vi "retrieve_graph_data.vi"(1 "Time":sgl, 2 "Data Cluster":T1, 3 "handle":i32) -> (0 "output cluster":T1)   [LabVIEW 2015]
uses:
  MWT.dll
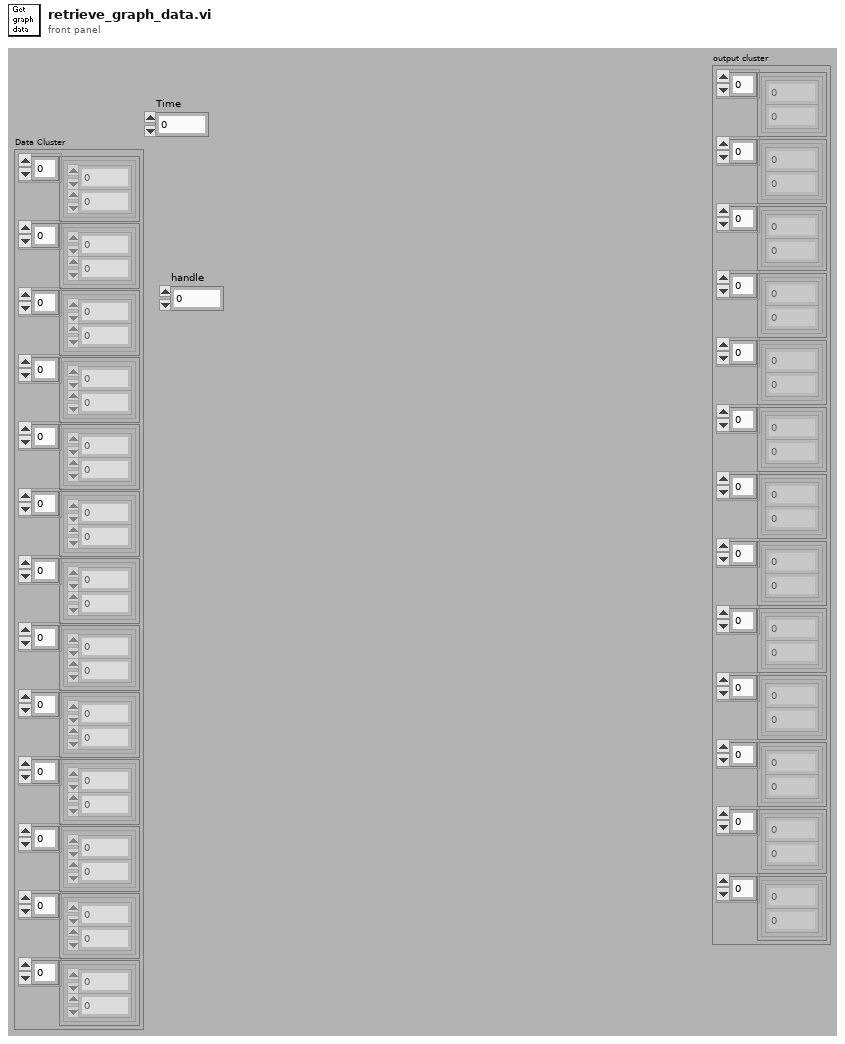
[diagram p1: front panel]
types:
  T1 = cluster{cluster{sgl, sgl}[], cluster{sgl, sgl}[], cluster{sgl, sgl}[], cluster{sgl, sgl}[], cluster{sgl, sgl}[], cluster{sgl, sgl}[], cluster{sgl, sgl}[], cluster{sgl, sgl}[], cluster{sgl, sgl}[], cluster{sgl, sgl}[], cluster{sgl, sgl}[], cluster{sgl, sgl}[], cluster{sgl, sgl}[]}
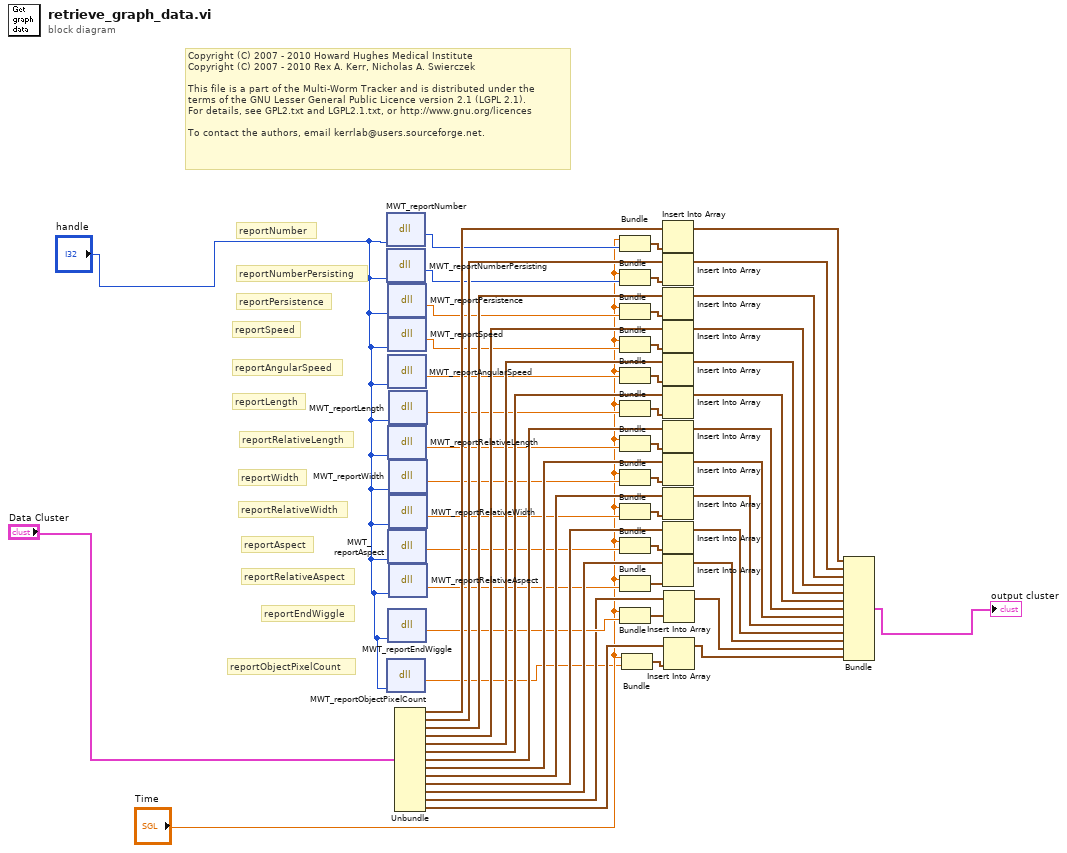
[diagram p0: block diagram]
diagram:
  # "reportObjectPixelCount"
  # "Copyright (C) 2007 - 2010 Howard Hughes Medical Institute\nCopyright (C) 2007 - 2010 Rex A. Kerr, Nicholas A. Swierczek\n \nThis file is a part of the Multi-Worm Tracker and is distributed under the\nterms of the GNU Lesser General Public Licence version 2.1 (LGPL 2.1).\nFor details, see GPL2.txt and LGPL2.1.txt, or http://www.gnu.org/licences\n \nTo contact the authors, email kerrlab@users.sourceforge.net."
  # "reportEndWiggle"
  # "reportRelativeAspect"
  # "reportAspect"
  # "reportRelativeWidth"
  # "reportWidth"
  # "reportRelativeLength"
  # "reportLength"
  # "reportAngularSpeed"
  # "reportSpeed"
  # "reportPersistence"
  # "reportNumberPersisting"
  # "reportNumber"
  n1 = dll-call lib="C:/Users/ramasamyl/Desktop/MWT/MWT.dll" fn="MWT_reportNumber"("handle"="handle") -> ("return type"=w12:i32)  [unwired: 4 in, 2 out]
  n2 = dll-call lib="C:/Users/ramasamyl/Desktop/MWT/MWT.dll" fn="MWT_reportNumberPersisting"("handle"="handle") -> ("return type"=w13:i32)  [unwired: 4 in, 2 out]
  n3 = dll-call lib="C:/Users/ramasamyl/Desktop/MWT/MWT.dll" fn="MWT_reportObjectPixelCount"("handle"="handle") -> ("return type"=w1:sgl)  [unwired: 4 in, 2 out]
  n4 = dll-call lib="C:/Users/ramasamyl/Desktop/MWT/MWT.dll" fn="MWT_reportPersistence"("handle"="handle") -> ("return type"=w14:sgl)  [unwired: 4 in, 2 out]
  n5 = dll-call lib="C:/Users/ramasamyl/Desktop/MWT/MWT.dll" fn="MWT_reportSpeed"("handle"="handle") -> ("return type"=w15:sgl)  [unwired: 4 in, 2 out]
  n6 = dll-call lib="C:/Users/ramasamyl/Desktop/MWT/MWT.dll" fn="MWT_reportAngularSpeed"("handle"="handle") -> ("return type"=w16:sgl)  [unwired: 4 in, 2 out]
  n7 = dll-call lib="C:/Users/ramasamyl/Desktop/MWT/MWT.dll" fn="MWT_reportRelativeLength"("handle"="handle") -> ("return type"=w18:sgl)  [unwired: 4 in, 2 out]
  n8 = dll-call lib="C:/Users/ramasamyl/Desktop/MWT/MWT.dll" fn="MWT_reportAspect"("handle"="handle") -> ("return type"=w21:sgl)  [unwired: 4 in, 2 out]
  n9 = dll-call lib="C:/Users/ramasamyl/Desktop/MWT/MWT.dll" fn="MWT_reportEndWiggle"("handle"="handle") -> ("return type"=w10:sgl)  [unwired: 4 in, 2 out]
  n10 = dll-call lib="C:/Users/ramasamyl/Desktop/MWT/MWT.dll" fn="MWT_reportLength"("handle"="handle") -> ("return type"=w17:sgl)  [unwired: 4 in, 2 out]
  n11 = dll-call lib="C:/Users/ramasamyl/Desktop/MWT/MWT.dll" fn="MWT_reportWidth"("handle"="handle") -> ("return type"=w19:sgl)  [unwired: 4 in, 2 out]
  n12 = dll-call lib="C:/Users/ramasamyl/Desktop/MWT/MWT.dll" fn="MWT_reportRelativeWidth"("handle"="handle") -> ("return type"=w20:sgl)  [unwired: 4 in, 2 out]
  n13 = dll-call lib="C:/Users/ramasamyl/Desktop/MWT/MWT.dll" fn="MWT_reportRelativeAspect"("handle"="handle") -> ("return type"=w22:sgl)  [unwired: 4 in, 2 out]
  n14 = Unbundle("Data Cluster") -> (w56:cluster{sgl, sgl}[], w55:cluster{sgl, sgl}[], w54:cluster{sgl, sgl}[], w53:cluster{sgl, sgl}[], w52:cluster{sgl, sgl}[], w51:cluster{sgl, sgl}[], w50:cluster{sgl, sgl}[], w49:cluster{sgl, sgl}[], w48:cluster{sgl, sgl}[], w47:cluster{sgl, sgl}[], w46:cluster{sgl, sgl}[], w8:cluster{sgl, sgl}[], w5:cluster{sgl, sgl}[])
  n15 = Bundle("Time"="Time", "return type"=w12) -> (w36:cluster{"Time":sgl, "return type":i32})  [unwired: 1 in]
  n16 = Bundle("Time"="Time", "return type"=w13) -> (w37:cluster{"Time":sgl, "return type":i32})  [unwired: 1 in]
  n17 = Bundle("Time"="Time", "return type"=w14) -> (w38:cluster{"Time":sgl, "return type":sgl})  [unwired: 1 in]
  n18 = Bundle("Time"="Time", "return type"=w15) -> (w39:cluster{"Time":sgl, "return type":sgl})  [unwired: 1 in]
  n19 = Bundle("Time"="Time", "return type"=w16) -> (w40:cluster{"Time":sgl, "return type":sgl})  [unwired: 1 in]
  n20 = Bundle("Time"="Time", "return type"=w17) -> (w41:cluster{"Time":sgl, "return type":sgl})  [unwired: 1 in]
  n21 = Bundle("Time"="Time", "return type"=w18) -> (w42:cluster{"Time":sgl, "return type":sgl})  [unwired: 1 in]
  n22 = Bundle("Time"="Time", "return type"=w19) -> (w43:cluster{"Time":sgl, "return type":sgl})  [unwired: 1 in]
  n23 = Bundle("Time"="Time", "return type"=w20) -> (w23:cluster{"Time":sgl, "return type":sgl})  [unwired: 1 in]
  n24 = Bundle("Time"="Time", "return type"=w21) -> (w44:cluster{"Time":sgl, "return type":sgl})  [unwired: 1 in]
  n25 = Bundle("Time"="Time", "return type"=w22) -> (w45:cluster{"Time":sgl, "return type":sgl})  [unwired: 1 in]
  n26 = Bundle("Time"="Time", "return type"=w10) -> (w11:cluster{"Time":sgl, "return type":sgl})  [unwired: 1 in]
  n27 = Bundle("Time"="Time", "return type"=w1) -> (w4:cluster{"Time":sgl, "return type":sgl})  [unwired: 1 in]
  n28 = Insert Into Array(array=w56, new element=w36) -> (w35:cluster{sgl, sgl}[])  [unwired: 1 in]
  n29 = Insert Into Array(array=w55, new element=w37) -> (w34:cluster{sgl, sgl}[])  [unwired: 1 in]
  n30 = Insert Into Array(array=w54, new element=w38) -> (w33:cluster{sgl, sgl}[])  [unwired: 1 in]
  n31 = Insert Into Array(array=w53, new element=w39) -> (w32:cluster{sgl, sgl}[])  [unwired: 1 in]
  n32 = Insert Into Array(array=w52, new element=w40) -> (w31:cluster{sgl, sgl}[])  [unwired: 1 in]
  n33 = Insert Into Array(array=w51, new element=w41) -> (w30:cluster{sgl, sgl}[])  [unwired: 1 in]
  n34 = Insert Into Array(array=w50, new element=w42) -> (w29:cluster{sgl, sgl}[])  [unwired: 1 in]
  n35 = Insert Into Array(array=w49, new element=w43) -> (w28:cluster{sgl, sgl}[])  [unwired: 1 in]
  n36 = Insert Into Array(array=w48, new element=w23) -> (w27:cluster{sgl, sgl}[])  [unwired: 1 in]
  n37 = Insert Into Array(array=w47, new element=w44) -> (w26:cluster{sgl, sgl}[])  [unwired: 1 in]
  n38 = Insert Into Array(array=w46, new element=w45) -> (w25:cluster{sgl, sgl}[])  [unwired: 1 in]
  n39 = Insert Into Array(array=w8, new element=w11) -> (w9:cluster{sgl, sgl}[])  [unwired: 1 in]
  n40 = Insert Into Array(array=w5, new element=w4) -> (w6:cluster{sgl, sgl}[])  [unwired: 1 in]
  n41 = Bundle(w35, w34, w33, w32, w31, w30, w29, w28, w27, w26, w25, w9, w6) -> (→"output cluster":T1)  [unwired: 1 in]
